vi "Get Current Step.vi"(8 "error in (no error)":errorcluster, 11 "Recipe in":refnum<class "Recipe.lvclass">) -> (0 "error out":errorcluster, 2 "Recipe Step":refnum<class "Recipe Step.lvclass">, 3 "Recipe out":refnum<class "Recipe.lvclass">)   [LabVIEW 2024, in "Recipe.lvclass"]
uses:
  Recipe.lvclass
  Recipe Step/Recipe Step.lvclass
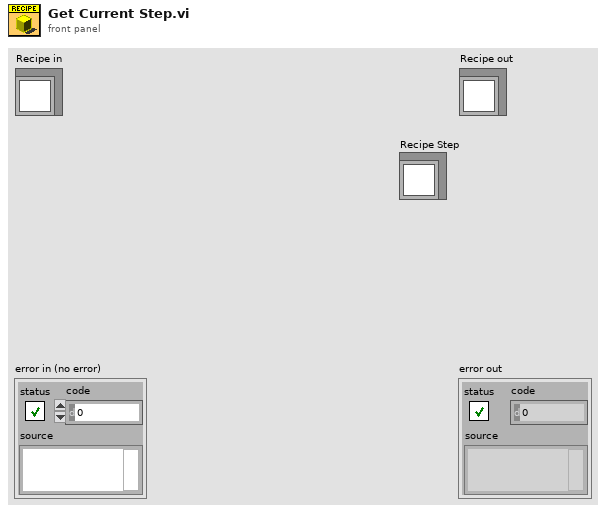
[diagram p1: front panel]
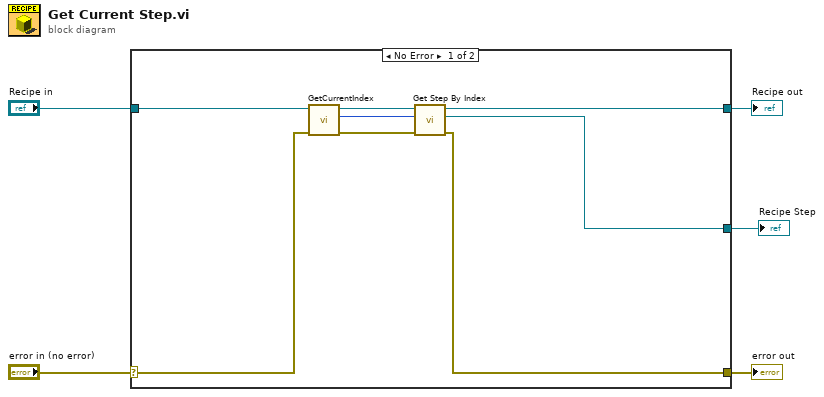
[diagram p0: block diagram]
diagram:
  n1 = case shown="No Error" "error in (no error)" {
    selector: "error in (no error)" -> [w11 w15]
    tunnel: [w12 w15] -> w4
    tunnel: [w13 w14] -> w2
    tunnel: "Recipe in" -> [w9 w14]
    tunnel: [w6 _] -> w1
    frame No Error {
      n2 = call-dynamic "GetCurrentIndex.vi"("Error In"=w11, "reference in"=w9) -> ("Error Out"=w10:errorcluster, "Current Index"=w7:u64, "reference out"=w8:refnum<class "Recipe.lvclass">)  [unwired: 7 in]
      n3 = call-dynamic "Get Step By Index.vi"("error in (no error)"=w10, "Index"=w7, "Recipe in"=w8) -> ("error out"=w12:errorcluster, "Recipe Step"=w6:refnum<class "Recipe Step.lvclass">, "Recipe out"=w13:refnum<class "Recipe.lvclass">)  [unwired: 6 in]
    }
    frame Error {
    }
  }
  "error out" <- w4
  "Recipe out" <- w2
  "Recipe Step" <- w1
